vi "Preset TIME JUDGment.vi"(8 "error in (no error)":errorcluster, 10 "Time [s]":dbl=0.3 min=0.3 max=99.9 step=0.1, 11 "VISA resource in":refnum<visa-resource-name>) -> (0 "error out":errorcluster, 3 "VISA resource out":refnum<visa-resource-name>)   [LabVIEW 2025, in "Chroma 19572.lvlib"]
doc: "This VI writes to the instrument the RAMP JUDG. state."
uses:
  <instrlib>/Chroma 19572/Chroma 19572.lvlib
panel:
  # "PreSet Time JUDGMENT"
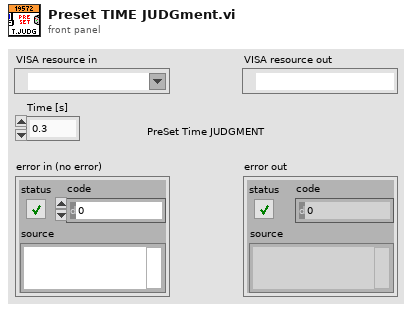
[diagram p1: front panel]
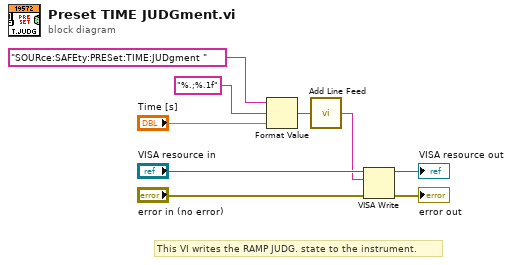
[diagram p0: block diagram]
diagram:
  # "This VI writes the RAMP JUDG. state to the instrument."
  n1 = Format Value(string ("")="SOURce:SAFEty:PRESet:TIME:JUDgment ", format string="%.;%.1f", value (0)="Time [s]") -> (output string=w3:string)
  n2 = call <instrlib>:"Add Line Feed.vi"("Command string"=w3) -> ("Concatenated string"=w1:string)  [unwired: 4 in]
  n3 = VISA Write(VISA resource name="VISA resource in", write buffer=w1, error in (no error)="error in (no error)") -> (VISA resource name out=→"VISA resource out":refnum<visa-resource-name>, error out=→"error out":errorcluster)  [unwired: 1 out]
